vi "Compare_Two_Term_Heirarchy.vi"   [LabVIEW 2021]
uses:
  Support/Compare/Two Term/SGL/AbsComp_Two Term_SGL.lvclass
  Support/Compare/Two Term/DBL/AbsComp_Two Term_DBL.lvclass
  Support/Compare/Two Term/EXT/AbsComp_Two Term_EXT.lvclass
  Support/Compare/Two Term/CPLX_DBL/AbsComp_Two Term_CPLX_DBL.lvclass
  Support/Compare/Two Term/CPLX_EXT/AbsComp_Two Term_CPLX_EXT.lvclass
  Support/Compare/Two Term/CPLX_SGL/AbsComp_Two Term_CPLX_SGL.lvclass
  Support/Compare/Two Term/I8/AbsComp_Two Term_I8.lvclass
  Support/Compare/Two Term/I16/AbsComp_Two Term_I16.lvclass
  Support/Compare/Two Term/I32/AbsComp_Two Term_I32.lvclass
  Support/Compare/Two Term/I64/AbsComp_Two Term_I64.lvclass
  Support/Compare/Two Term/U8/AbsComp_Two Term_U8.lvclass
  Support/Compare/Two Term/U16/AbsComp_Two Term_U16.lvclass
  Support/Compare/Two Term/U32/AbsComp_Two Term_U32.lvclass
  Support/Compare/Two Term/U64/AbsComp_Two Term_U64.lvclass
  Support/Equal/DBL/Equal_DBL.lvclass
  Support/Not Equal/DBL/Not Equal_DBL.lvclass
  Support/Greater/DBL/Greater_DBL.lvclass
  Support/Less/DBL/Less_DBL.lvclass
  Support/Greater Equal/DBL/Greater Equal_DBL.lvclass
  Support/Less Equal/DBL/Less Equal_DBL.lvclass
  Support/Equal/SGL/Equal_SGL.lvclass
  Support/Equal/EXT/Equal_EXT.lvclass
  Support/Equal/CPLX_DBL/Equal_CPLX_DBL.lvclass
  Support/Equal/CPLX_EXT/Equal_CPLX_EXT.lvclass
  Support/Equal/CPLX_SGL/Equal_CPLX_SGL.lvclass
  Support/Equal/I8/Equal_I8.lvclass
  Support/Equal/I16/Equal_I16.lvclass
  Support/Equal/I32/Equal_I32.lvclass
  Support/Equal/I64/Equal_I64.lvclass
  Support/Equal/U8/Equal_U8.lvclass
  Support/Equal/U16/Equal_U16.lvclass
  Support/Equal/U32/Equal_U32.lvclass
  Support/Equal/U64/Equal_U64.lvclass
  Support/Not Equal/SGL/Not Equal_SGL.lvclass
  Support/Not Equal/EXT/Not Equal_EXT.lvclass
  Support/Not Equal/CPLX_SGL/Not Equal_CPLX_SGL.lvclass
  Support/Not Equal/CPLX_DBL/Not Equal_CPLX_DBL.lvclass
  Support/Not Equal/CPLX_EXT/Not Equal_CPLX_EXT.lvclass
  Support/Not Equal/I8/Not Equal_I8.lvclass
  Support/Not Equal/I16/Not Equal_I16.lvclass
  Support/Not Equal/I32/Not Equal_I32.lvclass
  Support/Not Equal/I64/Not Equal_I64.lvclass
  Support/Not Equal/U8/Not Equal_U8.lvclass
  Support/Not Equal/U16/Not Equal_U16.lvclass
  Support/Not Equal/U32/Not Equal_U32.lvclass
  Support/Not Equal/U64/Not Equal_U64.lvclass
  Support/Greater/SGL/Greater_SGL.lvclass
  Support/Greater/EXT/Greater_EXT.lvclass
  Support/Greater/I8/Greater_I8.lvclass
  Support/Greater/I16/Greater_I16.lvclass
  Support/Greater/I32/Greater_I32.lvclass
  Support/Greater/I64/Greater_I64.lvclass
  Support/Greater/U8/Greater_U8.lvclass
  Support/Greater/U16/Greater_U16.lvclass
  Support/Greater/U32/Greater_U32.lvclass
  Support/Greater/U64/Greater_U64.lvclass
  Support/Less/SGL/Less_SGL.lvclass
  Support/Less/EXT/Less_EXT.lvclass
  Support/Less/I8/Less_I8.lvclass
  Support/Less/I16/Less_I16.lvclass
  Support/Less/I32/Less_I32.lvclass
  Support/Less/I64/Less_I64.lvclass
  Support/Less/U8/Less_U8.lvclass
  Support/Less/U16/Less_U16.lvclass
  Support/Less/U32/Less_U32.lvclass
  Support/Less/U64/Less_U64.lvclass
  Support/Greater Equal/SGL/Greater Equal_SGL.lvclass
  Support/Greater Equal/EXT/Greater Equal_EXT.lvclass
  Support/Greater Equal/I8/Greater Equal_I8.lvclass
  Support/Greater Equal/I16/Greater Equal_I16.lvclass
  Support/Greater Equal/I32/Greater Equal_I32.lvclass
  Support/Greater Equal/I64/Greater Equal_I64.lvclass
  Support/Greater Equal/U8/Greater Equal_U8.lvclass
  Support/Greater Equal/U16/Greater Equal_U16.lvclass
  Support/Greater Equal/U32/Greater Equal_U32.lvclass
  Support/Greater Equal/U64/Greater Equal_U64.lvclass
  Support/Less Equal/SGL/Less Equal_SGL.lvclass
  Support/Less Equal/EXT/Less Equal_EXT.lvclass
  Support/Less Equal/I8/Less Equal_I8.lvclass
  Support/Less Equal/I16/Less Equal_I16.lvclass
  Support/Less Equal/I32/Less Equal_I32.lvclass
  Support/Less Equal/I64/Less Equal_I64.lvclass
  Support/Less Equal/U8/Less Equal_U8.lvclass
  Support/Less Equal/U16/Less Equal_U16.lvclass
  Support/Less Equal/U32/Less Equal_U32.lvclass
  Support/Less Equal/U64/Less Equal_U64.lvclass
  Support/Equal/STR/Equal_STR.lvclass
  Support/Greater/Time/Greater_Time.lvclass
  Support/Less/Time/Less_Time.lvclass
  Support/Greater Equal/Time/Greater Equal_Time.lvclass
  Support/Less Equal/Time/Less Equal_Time.lvclass
  Support/Equal/Time/Equal_Time.lvclass
  Support/Not Equal/Time/Not Equal_Time.lvclass
  Support/Not Equal/STR/Not Equal_STR.lvclass
  Support/Compare/Two Term/Time/AbsComp_Two Term_Time.lvclass
  Support/Compare/Two Term/STR/AbsComp_Two Term_STR.lvclass
panel:
  # "SEE DIAGRAM\nFOR Hierarchy"
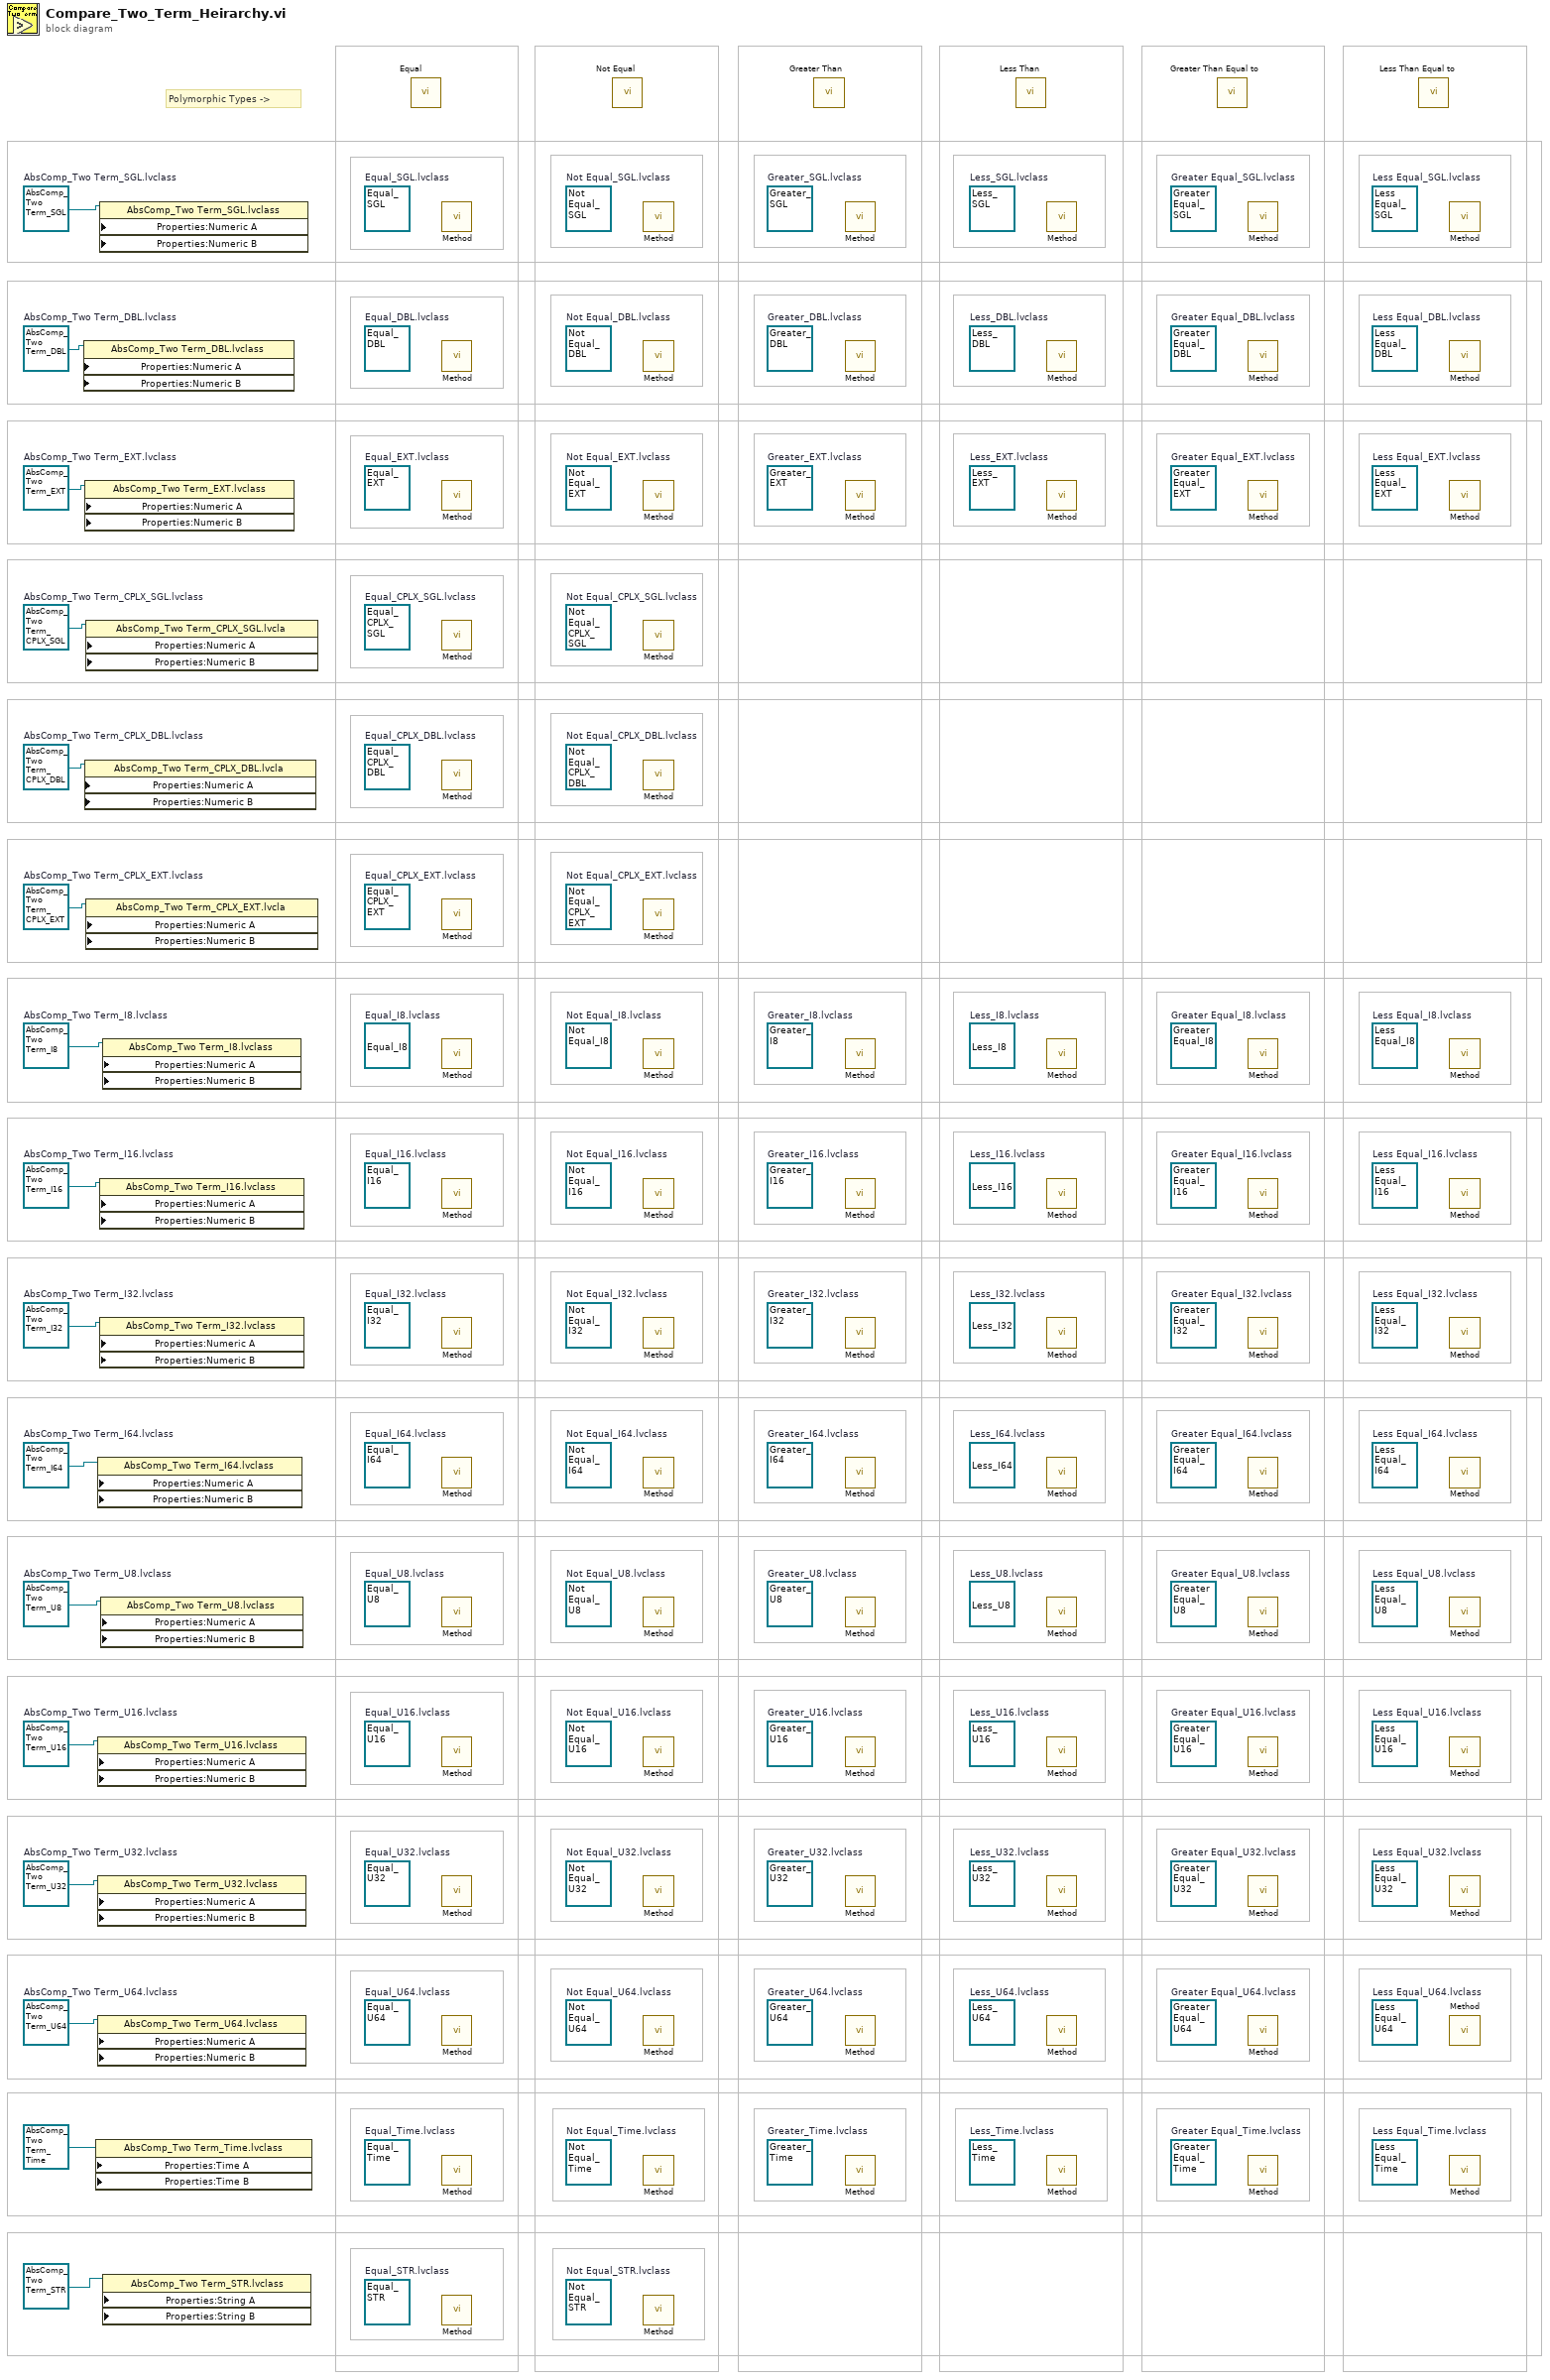
[diagram p0: block diagram]
diagram:
  (unwired) refnum<class "Not Equal_STR.lvclass"> refnum  # Not Equal_STR.lvclass
  (unwired) refnum<class "Equal_STR.lvclass"> refnum  # Equal_STR.lvclass
  (unwired) refnum<class "Less Equal_Time.lvclass"> refnum  # Less Equal_Time.lvclass
  (unwired) refnum<class "Greater Equal_Time.lvclass"> refnum  # Greater Equal_Time.lvclass
  (unwired) refnum<class "Less_Time.lvclass"> refnum  # Less_Time.lvclass
  (unwired) refnum<class "Greater_Time.lvclass"> refnum  # Greater_Time.lvclass
  (unwired) refnum<class "Not Equal_Time.lvclass"> refnum  # Not Equal_Time.lvclass
  (unwired) refnum<class "Equal_Time.lvclass"> refnum  # Equal_Time.lvclass
  (unwired) refnum<class "Less Equal_U64.lvclass"> refnum  # Less Equal_U64.lvclass
  (unwired) refnum<class "Less Equal_U32.lvclass"> refnum  # Less Equal_U32.lvclass
  (unwired) refnum<class "Less Equal_U16.lvclass"> refnum  # Less Equal_U16.lvclass
  (unwired) refnum<class "Less Equal_U8.lvclass"> refnum  # Less Equal_U8.lvclass
  (unwired) refnum<class "Less Equal_I64.lvclass"> refnum  # Less Equal_I64.lvclass
  (unwired) refnum<class "Less Equal_I32.lvclass"> refnum  # Less Equal_I32.lvclass
  (unwired) refnum<class "Less Equal_I16.lvclass"> refnum  # Less Equal_I16.lvclass
  (unwired) refnum<class "Less Equal_I8.lvclass"> refnum  # Less Equal_I8.lvclass
  (unwired) refnum<class "Less Equal_EXT.lvclass"> refnum  # Less Equal_EXT.lvclass
  (unwired) refnum<class "Less Equal_DBL.lvclass"> refnum  # Less Equal_DBL.lvclass
  (unwired) refnum<class "Less Equal_SGL.lvclass"> refnum  # Less Equal_SGL.lvclass
  (unwired) refnum<class "Greater Equal_U64.lvclass"> refnum  # Greater Equal_U64.lvclass
  (unwired) refnum<class "Greater Equal_U32.lvclass"> refnum  # Greater Equal_U32.lvclass
  (unwired) refnum<class "Greater Equal_U16.lvclass"> refnum  # Greater Equal_U16.lvclass
  (unwired) refnum<class "Greater Equal_U8.lvclass"> refnum  # Greater Equal_U8.lvclass
  (unwired) refnum<class "Greater Equal_I64.lvclass"> refnum  # Greater Equal_I64.lvclass
  (unwired) refnum<class "Greater Equal_I32.lvclass"> refnum  # Greater Equal_I32.lvclass
  (unwired) refnum<class "Greater Equal_I16.lvclass"> refnum  # Greater Equal_I16.lvclass
  (unwired) refnum<class "Greater Equal_I8.lvclass"> refnum  # Greater Equal_I8.lvclass
  (unwired) refnum<class "Greater Equal_EXT.lvclass"> refnum  # Greater Equal_EXT.lvclass
  (unwired) refnum<class "Greater Equal_DBL.lvclass"> refnum  # Greater Equal_DBL.lvclass
  (unwired) refnum<class "Greater Equal_SGL.lvclass"> refnum  # Greater Equal_SGL.lvclass
  (unwired) refnum<class "Less_U64.lvclass"> refnum  # Less_U64.lvclass
  (unwired) refnum<class "Less_U32.lvclass"> refnum  # Less_U32.lvclass
  (unwired) refnum<class "Less_U16.lvclass"> refnum  # Less_U16.lvclass
  (unwired) refnum<class "Less_U8.lvclass"> refnum  # Less_U8.lvclass
  (unwired) refnum<class "Less_I64.lvclass"> refnum  # Less_I64.lvclass
  (unwired) refnum<class "Less_I32.lvclass"> refnum  # Less_I32.lvclass
  (unwired) refnum<class "Less_I16.lvclass"> refnum  # Less_I16.lvclass
  (unwired) refnum<class "Less_I8.lvclass"> refnum  # Less_I8.lvclass
  (unwired) refnum<class "Less_EXT.lvclass"> refnum  # Less_EXT.lvclass
  (unwired) refnum<class "Less_DBL.lvclass"> refnum  # Less_DBL.lvclass
  (unwired) refnum<class "Less_SGL.lvclass"> refnum  # Less_SGL.lvclass
  (unwired) refnum<class "Greater_U64.lvclass"> refnum  # Greater_U64.lvclass
  (unwired) refnum<class "Greater_U32.lvclass"> refnum  # Greater_U32.lvclass
  (unwired) refnum<class "Greater_U16.lvclass"> refnum  # Greater_U16.lvclass
  (unwired) refnum<class "Greater_U8.lvclass"> refnum  # Greater_U8.lvclass
  (unwired) refnum<class "Greater_I64.lvclass"> refnum  # Greater_I64.lvclass
  (unwired) refnum<class "Greater_I32.lvclass"> refnum  # Greater_I32.lvclass
  (unwired) refnum<class "Greater_I16.lvclass"> refnum  # Greater_I16.lvclass
  (unwired) refnum<class "Greater_I8.lvclass"> refnum  # Greater_I8.lvclass
  (unwired) refnum<class "Greater_EXT.lvclass"> refnum  # Greater_EXT.lvclass
  (unwired) refnum<class "Greater_DBL.lvclass"> refnum  # Greater_DBL.lvclass
  (unwired) refnum<class "Greater_SGL.lvclass"> refnum  # Greater_SGL.lvclass
  (unwired) refnum<class "Not Equal_U64.lvclass"> refnum  # Not Equal_U64.lvclass
  (unwired) refnum<class "Not Equal_U32.lvclass"> refnum  # Not Equal_U32.lvclass
  (unwired) refnum<class "Not Equal_U16.lvclass"> refnum  # Not Equal_U16.lvclass
  (unwired) refnum<class "Not Equal_U8.lvclass"> refnum  # Not Equal_U8.lvclass
  (unwired) refnum<class "Not Equal_I64.lvclass"> refnum  # Not Equal_I64.lvclass
  (unwired) refnum<class "Not Equal_I32.lvclass"> refnum  # Not Equal_I32.lvclass
  (unwired) refnum<class "Not Equal_I16.lvclass"> refnum  # Not Equal_I16.lvclass
  (unwired) refnum<class "Not Equal_I8.lvclass"> refnum  # Not Equal_I8.lvclass
  (unwired) refnum<class "Not Equal_CPLX_EXT.lvclass"> refnum  # Not Equal_CPLX_EXT.lvclass
  (unwired) refnum<class "Not Equal_CPLX_DBL.lvclass"> refnum  # Not Equal_CPLX_DBL.lvclass
  (unwired) refnum<class "Not Equal_CPLX_SGL.lvclass"> refnum  # Not Equal_CPLX_SGL.lvclass
  (unwired) refnum<class "Not Equal_EXT.lvclass"> refnum  # Not Equal_EXT.lvclass
  (unwired) refnum<class "Not Equal_DBL.lvclass"> refnum  # Not Equal_DBL.lvclass
  (unwired) refnum<class "Not Equal_SGL.lvclass"> refnum  # Not Equal_SGL.lvclass
  (unwired) refnum<class "Equal_U64.lvclass"> refnum  # Equal_U64.lvclass
  (unwired) refnum<class "Equal_U32.lvclass"> refnum  # Equal_U32.lvclass
  (unwired) refnum<class "Equal_U16.lvclass"> refnum  # Equal_U16.lvclass
  (unwired) refnum<class "Equal_U8.lvclass"> refnum  # Equal_U8.lvclass
  (unwired) refnum<class "Equal_I64.lvclass"> refnum  # Equal_I64.lvclass
  (unwired) refnum<class "Equal_I32.lvclass"> refnum  # Equal_I32.lvclass
  (unwired) refnum<class "Equal_I16.lvclass"> refnum  # Equal_I16.lvclass
  (unwired) refnum<class "Equal_I8.lvclass"> refnum  # Equal_I8.lvclass
  (unwired) refnum<class "Equal_CPLX_SGL.lvclass"> refnum  # Equal_CPLX_SGL.lvclass
  (unwired) refnum<class "Equal_CPLX_DBL.lvclass"> refnum  # Equal_CPLX_DBL.lvclass
  (unwired) refnum<class "Equal_CPLX_EXT.lvclass"> refnum  # Equal_CPLX_EXT.lvclass
  (unwired) refnum<class "Equal_EXT.lvclass"> refnum  # Equal_EXT.lvclass
  (unwired) refnum<class "Equal_DBL.lvclass"> refnum  # Equal_DBL.lvclass
  (unwired) refnum<class "Equal_SGL.lvclass"> refnum  # Equal_SGL.lvclass
  w15 = refnum<class "AbsComp_Two Term_U64.lvclass"> refnum  # AbsComp_Two Term_U64.lvclass
  w14 = refnum<class "AbsComp_Two Term_U32.lvclass"> refnum  # AbsComp_Two Term_U32.lvclass
  w13 = refnum<class "AbsComp_Two Term_U16.lvclass"> refnum  # AbsComp_Two Term_U16.lvclass
  w12 = refnum<class "AbsComp_Two Term_U8.lvclass"> refnum  # AbsComp_Two Term_U8.lvclass
  w11 = refnum<class "AbsComp_Two Term_I64.lvclass"> refnum  # AbsComp_Two Term_I64.lvclass
  w10 = refnum<class "AbsComp_Two Term_I32.lvclass"> refnum  # AbsComp_Two Term_I32.lvclass
  w9 = refnum<class "AbsComp_Two Term_I16.lvclass"> refnum  # AbsComp_Two Term_I16.lvclass
  w8 = refnum<class "AbsComp_Two Term_I8.lvclass"> refnum  # AbsComp_Two Term_I8.lvclass
  w5 = refnum<class "AbsComp_Two Term_CPLX_SGL.lvclass"> refnum  # AbsComp_Two Term_CPLX_SGL.lvclass
  w3 = refnum<class "AbsComp_Two Term_CPLX_EXT.lvclass"> refnum  # AbsComp_Two Term_CPLX_EXT.lvclass
  w4 = refnum<class "AbsComp_Two Term_CPLX_DBL.lvclass"> refnum  # AbsComp_Two Term_CPLX_DBL.lvclass
  w7 = refnum<class "AbsComp_Two Term_EXT.lvclass"> refnum  # AbsComp_Two Term_EXT.lvclass
  w6 = refnum<class "AbsComp_Two Term_DBL.lvclass"> refnum  # AbsComp_Two Term_DBL.lvclass
  w16 = refnum<class "AbsComp_Two Term_SGL.lvclass"> refnum  # AbsComp_Two Term_SGL.lvclass
  # "Polymorphic Types ->"
  n1 = property class="AbsComp_Two Term_DBL.lvclass" props=["Properties:Numeric A", "Properties:Numeric B"](reference=w6) -> ()  [unwired: 3 in, 2 out]
  n2 = property class="AbsComp_Two Term_CPLX_DBL.lvcla" props=["Properties:Numeric A", "Properties:Numeric B"](reference=w4) -> ()  [unwired: 3 in, 2 out]
  n3 = property class="AbsComp_Two Term_EXT.lvclass" props=["Properties:Numeric A", "Properties:Numeric B"](reference=w7) -> ()  [unwired: 3 in, 2 out]
  n4 = property class="AbsComp_Two Term_CPLX_SGL.lvcla" props=["Properties:Numeric A", "Properties:Numeric B"](reference=w5) -> ()  [unwired: 3 in, 2 out]
  n5 = property class="AbsComp_Two Term_CPLX_EXT.lvcla" props=["Properties:Numeric A", "Properties:Numeric B"](reference=w3) -> ()  [unwired: 3 in, 2 out]
  n6 = property class="AbsComp_Two Term_Time.lvclass" props=["Properties:Time A", "Properties:Time B"](reference=refnum<class "AbsComp_Two Term_Time.lvclass"> refnum ("AbsComp_Two Term_Time.lvclass")) -> ()  [unwired: 3 in, 2 out]
  n7 = property class="AbsComp_Two Term_I64.lvclass" props=["Properties:Numeric A", "Properties:Numeric B"](reference=w11) -> ()  [unwired: 3 in, 2 out]
  n8 = property class="AbsComp_Two Term_U16.lvclass" props=["Properties:Numeric A", "Properties:Numeric B"](reference=w13) -> ()  [unwired: 3 in, 2 out]
  n9 = property class="AbsComp_Two Term_U32.lvclass" props=["Properties:Numeric A", "Properties:Numeric B"](reference=w14) -> ()  [unwired: 3 in, 2 out]
  n10 = property class="AbsComp_Two Term_U64.lvclass" props=["Properties:Numeric A", "Properties:Numeric B"](reference=w15) -> ()  [unwired: 3 in, 2 out]
  n11 = property class="AbsComp_Two Term_SGL.lvclass" props=["Properties:Numeric A", "Properties:Numeric B"](reference=w16) -> ()  [unwired: 3 in, 2 out]
  n12 = property class="AbsComp_Two Term_I16.lvclass" props=["Properties:Numeric A", "Properties:Numeric B"](reference=w9) -> ()  [unwired: 3 in, 2 out]
  n13 = property class="AbsComp_Two Term_I32.lvclass" props=["Properties:Numeric A", "Properties:Numeric B"](reference=w10) -> ()  [unwired: 3 in, 2 out]
  n14 = property class="AbsComp_Two Term_U8.lvclass" props=["Properties:Numeric A", "Properties:Numeric B"](reference=w12) -> ()  [unwired: 3 in, 2 out]
  n15 = property class="AbsComp_Two Term_I8.lvclass" props=["Properties:Numeric A", "Properties:Numeric B"](reference=w8) -> ()  [unwired: 3 in, 2 out]
  n16 = property class="AbsComp_Two Term_STR.lvclass" props=["Properties:String A", "Properties:String B"](reference=refnum<class "AbsComp_Two Term_STR.lvclass"> refnum ("AbsComp_Two Term_STR.lvclass")) -> ()  [unwired: 3 in, 2 out]
  n17 = call-poly "Equal.vi"() -> ()  [unwired: 6 in, 1 out]
  n18 = call "Method.vi"() -> ()  [unwired: 6 in, 1 out]
  n19 = call "Method.vi"() -> ()  [unwired: 6 in, 1 out]
  n20 = call "Method.vi"() -> ()  [unwired: 6 in, 1 out]
  n21 = call "Method.vi"() -> ()  [unwired: 6 in, 1 out]
  n22 = call "Method.vi"() -> ()  [unwired: 6 in, 1 out]
  n23 = call "Method.vi"() -> ()  [unwired: 6 in, 1 out]
  n24 = call "Method.vi"() -> ()  [unwired: 6 in, 1 out]
  n25 = call "Method.vi"() -> ()  [unwired: 6 in, 1 out]
  n26 = call "Method.vi"() -> ()  [unwired: 6 in, 1 out]
  n27 = call "Method.vi"() -> ()  [unwired: 6 in, 1 out]
  n28 = call "Method.vi"() -> ()  [unwired: 6 in, 1 out]
  n29 = call "Method.vi"() -> ()  [unwired: 6 in, 1 out]
  n30 = call "Method.vi"() -> ()  [unwired: 6 in, 1 out]
  n31 = call "Method.vi"() -> ()  [unwired: 6 in, 1 out]
  n32 = call "Method.vi"() -> ()  [unwired: 6 in, 1 out]
  n33 = call "Method.vi"() -> ()  [unwired: 6 in, 1 out]
  n34 = call-poly "Not Equal.vi"() -> ()  [unwired: 6 in, 1 out]
  n35 = call "Method.vi"() -> ()  [unwired: 6 in, 1 out]
  n36 = call "Method.vi"() -> ()  [unwired: 6 in, 1 out]
  n37 = call "Method.vi"() -> ()  [unwired: 6 in, 1 out]
  n38 = call "Method.vi"() -> ()  [unwired: 6 in, 1 out]
  n39 = call "Method.vi"() -> ()  [unwired: 6 in, 1 out]
  n40 = call "Method.vi"() -> ()  [unwired: 6 in, 1 out]
  n41 = call "Method.vi"() -> ()  [unwired: 6 in, 1 out]
  n42 = call "Method.vi"() -> ()  [unwired: 6 in, 1 out]
  n43 = call "Method.vi"() -> ()  [unwired: 6 in, 1 out]
  n44 = call "Method.vi"() -> ()  [unwired: 6 in, 1 out]
  n45 = call "Method.vi"() -> ()  [unwired: 6 in, 1 out]
  n46 = call "Method.vi"() -> ()  [unwired: 6 in, 1 out]
  n47 = call "Method.vi"() -> ()  [unwired: 6 in, 1 out]
  n48 = call "Method.vi"() -> ()  [unwired: 6 in, 1 out]
  n49 = call "Method.vi"() -> ()  [unwired: 6 in, 1 out]
  n50 = call "Method.vi"() -> ()  [unwired: 6 in, 1 out]
  n51 = call-poly "Greater Than.vi"() -> ()  [unwired: 6 in, 1 out]
  n52 = call "Method.vi"() -> ()  [unwired: 6 in, 1 out]
  n53 = call "Method.vi"() -> ()  [unwired: 6 in, 1 out]
  n54 = call "Method.vi"() -> ()  [unwired: 6 in, 1 out]
  n55 = call "Method.vi"() -> ()  [unwired: 6 in, 1 out]
  n56 = call "Method.vi"() -> ()  [unwired: 6 in, 1 out]
  n57 = call "Method.vi"() -> ()  [unwired: 6 in, 1 out]
  n58 = call "Method.vi"() -> ()  [unwired: 6 in, 1 out]
  n59 = call "Method.vi"() -> ()  [unwired: 6 in, 1 out]
  n60 = call "Method.vi"() -> ()  [unwired: 6 in, 1 out]
  n61 = call "Method.vi"() -> ()  [unwired: 6 in, 1 out]
  n62 = call "Method.vi"() -> ()  [unwired: 6 in, 1 out]
  n63 = call "Method.vi"() -> ()  [unwired: 6 in, 1 out]
  n64 = call-poly "Less Than.vi"() -> ()  [unwired: 6 in, 1 out]
  n65 = call "Method.vi"() -> ()  [unwired: 6 in, 1 out]
  n66 = call "Method.vi"() -> ()  [unwired: 6 in, 1 out]
  n67 = call "Method.vi"() -> ()  [unwired: 6 in, 1 out]
  n68 = call "Method.vi"() -> ()  [unwired: 6 in, 1 out]
  n69 = call "Method.vi"() -> ()  [unwired: 6 in, 1 out]
  n70 = call "Method.vi"() -> ()  [unwired: 6 in, 1 out]
  n71 = call "Method.vi"() -> ()  [unwired: 6 in, 1 out]
  n72 = call "Method.vi"() -> ()  [unwired: 6 in, 1 out]
  n73 = call "Method.vi"() -> ()  [unwired: 6 in, 1 out]
  n74 = call "Method.vi"() -> ()  [unwired: 6 in, 1 out]
  n75 = call "Method.vi"() -> ()  [unwired: 6 in, 1 out]
  n76 = call "Method.vi"() -> ()  [unwired: 6 in, 1 out]
  n77 = call-poly "Greater Than Equal to.vi"() -> ()  [unwired: 6 in, 1 out]
  n78 = call "Method.vi"() -> ()  [unwired: 6 in, 1 out]
  n79 = call "Method.vi"() -> ()  [unwired: 6 in, 1 out]
  n80 = call "Method.vi"() -> ()  [unwired: 6 in, 1 out]
  n81 = call "Method.vi"() -> ()  [unwired: 6 in, 1 out]
  n82 = call "Method.vi"() -> ()  [unwired: 6 in, 1 out]
  n83 = call "Method.vi"() -> ()  [unwired: 6 in, 1 out]
  n84 = call "Method.vi"() -> ()  [unwired: 6 in, 1 out]
  n85 = call "Method.vi"() -> ()  [unwired: 6 in, 1 out]
  n86 = call "Method.vi"() -> ()  [unwired: 6 in, 1 out]
  n87 = call "Method.vi"() -> ()  [unwired: 6 in, 1 out]
  n88 = call "Method.vi"() -> ()  [unwired: 6 in, 1 out]
  n89 = call "Method.vi"() -> ()  [unwired: 6 in, 1 out]
  n90 = call-poly "Less Than Equal to.vi"() -> ()  [unwired: 6 in, 1 out]
  n91 = call "Method.vi"() -> ()  [unwired: 6 in, 1 out]
  n92 = call "Method.vi"() -> ()  [unwired: 6 in, 1 out]
  n93 = call "Method.vi"() -> ()  [unwired: 6 in, 1 out]
  n94 = call "Method.vi"() -> ()  [unwired: 6 in, 1 out]
  n95 = call "Method.vi"() -> ()  [unwired: 6 in, 1 out]
  n96 = call "Method.vi"() -> ()  [unwired: 6 in, 1 out]
  n97 = call "Method.vi"() -> ()  [unwired: 6 in, 1 out]
  n98 = call "Method.vi"() -> ()  [unwired: 6 in, 1 out]
  n99 = call "Method.vi"() -> ()  [unwired: 6 in, 1 out]
  n100 = call "Method.vi"() -> ()  [unwired: 6 in, 1 out]
  n101 = call "Method.vi"() -> ()  [unwired: 6 in, 1 out]
  n102 = call "Method.vi"() -> ()  [unwired: 6 in, 1 out]
